vi "Logging Message Loop.vi"(8 "error in (no error)":errorcluster) -> (0 "error out":errorcluster)   [LabVIEW 2020, in "SAVE.lvlib"]
doc: "The message loop subVI to handle messages pertaining to logging data."
uses:
  SAVE.lvlib
  Test Driver/System Preset.ctl
  support/PCT FGV CMD.ctl
  Logging State.ctl
  Save Configuration.ctl
  support/Message Queue/Enqueue Message (Single).vi
  <vilib>/Utility/error.llb/Error Cluster From Error Code.vi
  <vilib>/ErrorRing/Error Ring.xnode
  support/Message Queue/Message Queue.lvlib
panel:
  out "Gage Config":T1(array[cluster])
  out "System Preset":T2 {"Test Configuration"."SP List" format="%#.1g"}
  # "X"
  # "Y"
  # "Cycles"
  # "Point Delay"
  # "Up"
  # "Down"
  # "Z Axes"
  # "#C"
  # "In"
  # "Out"
  # "Cleaning [sec]"
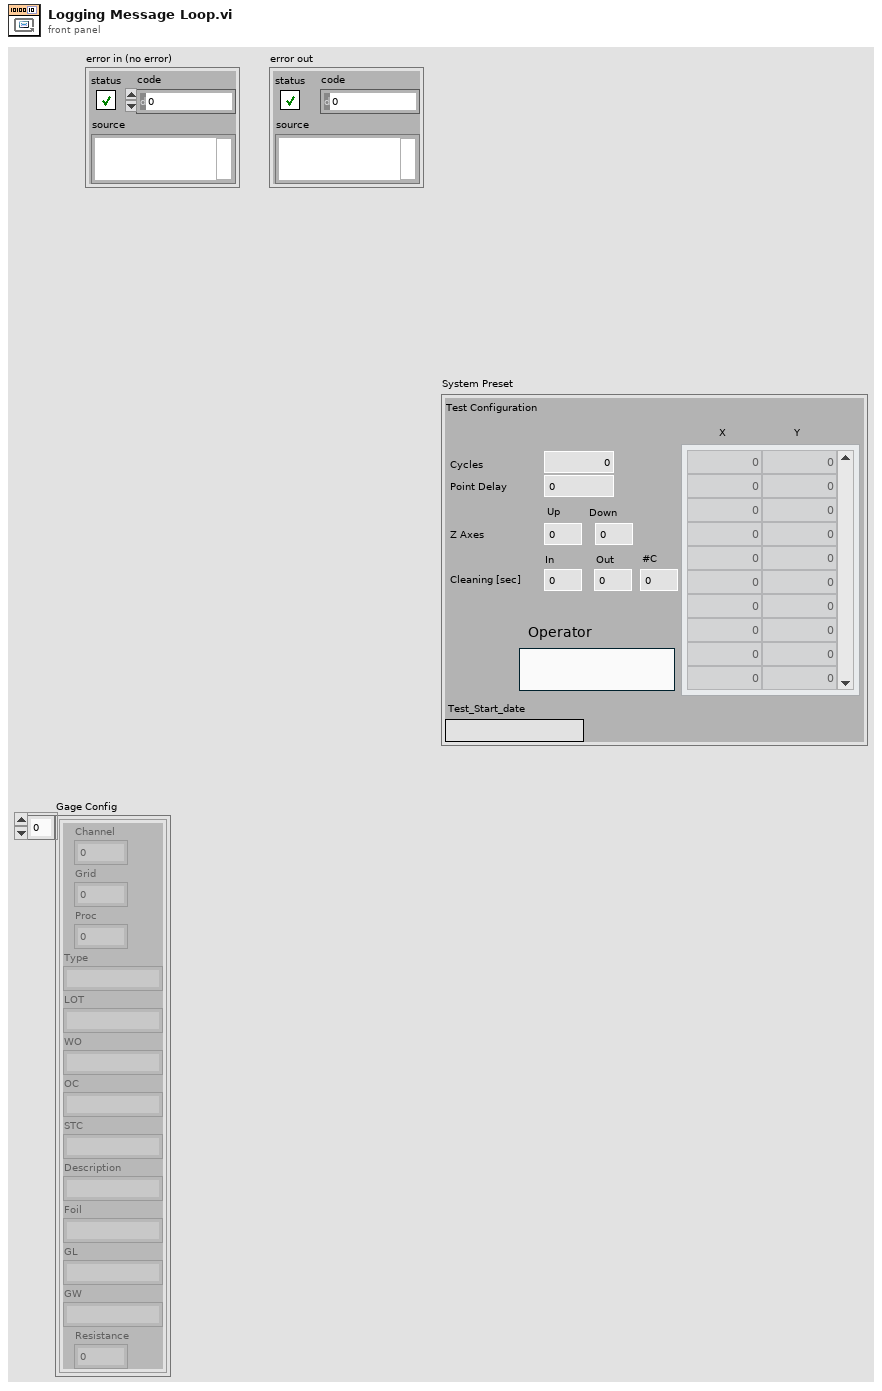
[diagram p1: front panel]
types:
  T1 = cluster{"Channel":u16, "Grid":u16, "Proc":u16, "Type":string, "LOT":string, "WO":string, "OC":string, "STC":string, "Description":string, "Foil":string, "GL":string, "GW":string, "Resistance":dbl}[]
  T2 = typedef "System Preset.ctl" = cluster{"Test Configuration":cluster{"Cycles":i32, "Z Up":dbl, "SP List":dbl[][], "Operator":string, "Point Delay":i32, "Z Up 2":dbl, "Cleaning In":dbl, "Cleaning Out":dbl, "Cleaning Cycles":i32}, "Test_Start_date":string}
  T3 = cluster{"Adhesive Type":string, "Adhesive LOT":string, "Calibration Date":string, "REF Gage Configuration":cluster{"Type":string, "Resistance":dbl, "LOT":string, "Replacement Date":string, "GF":dbl, "Ref Channel":dbl}, "Limits":cluster{"X_t":i32, "X_c":i32, "Exe_t":i32, "Exe_c":i32}, "Gage Config":cluster{"Channel":u16, "Grid":u16, "Proc":u16, "Type":string, "LOT":string, "WO":string, "OC":string, "STC":string, "Description":string, "Foil":string, "GL":string, "GW":string, "Resistance":dbl}[]}
  T4 = typedef "PCT FGV CMD.ctl" = enum16{"INIT", "GET", "SET"}
  T5 = typedef "Message Queue.lvlib/All Message Queues.ctl" = cluster{"UI":refnum<queue>, "Logging":refnum<queue>, "LOG":refnum<queue>, "ALARM":refnum<queue>, "Test":refnum<queue>, "Answer":refnum<queue>, "PLC":refnum<queue>, "DB":refnum<queue>, "Report":refnum<queue>, "OPC":refnum<queue>, "Procedure":refnum<queue>, "PalmSens":refnum<queue>, "SYS 7000 Reader":refnum<queue>, "SWITCH":refnum<queue>, "MOTOR":refnum<queue>, "MOTION":refnum<queue>, "HIDEN":refnum<queue>, "VALVE":refnum<queue>, "MFC":refnum<queue>, "PUMP IN":refnum<queue>, "PUMP OUT":refnum<queue>}
  T6 = typedef "PCT Data REFs.ctl" = cluster{"PLC AI Notifier":refnum<notifier>, "PS Data Queue":refnum<queue>, "BTN Queue":refnum<queue>, "PLC DI notifier":refnum<notifier>, "Timer notifier":refnum<notifier>, "DMM PS":refnum<notifier>, "DMM Gages":refnum<notifier>, "XYZ notifier":refnum<notifier>, "Test Notifier":refnum<notifier>, "Scanner notifier":refnum<notifier>, "OPC Notifier":refnum<notifier>, "HIDEN queue":refnum<queue>}
  T7 = typedef "SAVE.lvlib/Save Configuration.ctl" = cluster{"Log File Base Path":path, "TDMS File Reference":refnum<k34>, "Reset":bool, "Wait":dbl, "Start Time":dbl, "Update Rate":u16, "Channel Names":string[], "System Preset":variant}
  T8 = typedef "SAVE.lvlib/Logging State.ctl" = enum16{"Idle", "Logging"}
  T9 = enum16{"open", "open or create", "create or replace", "create", "open (read-only)"}
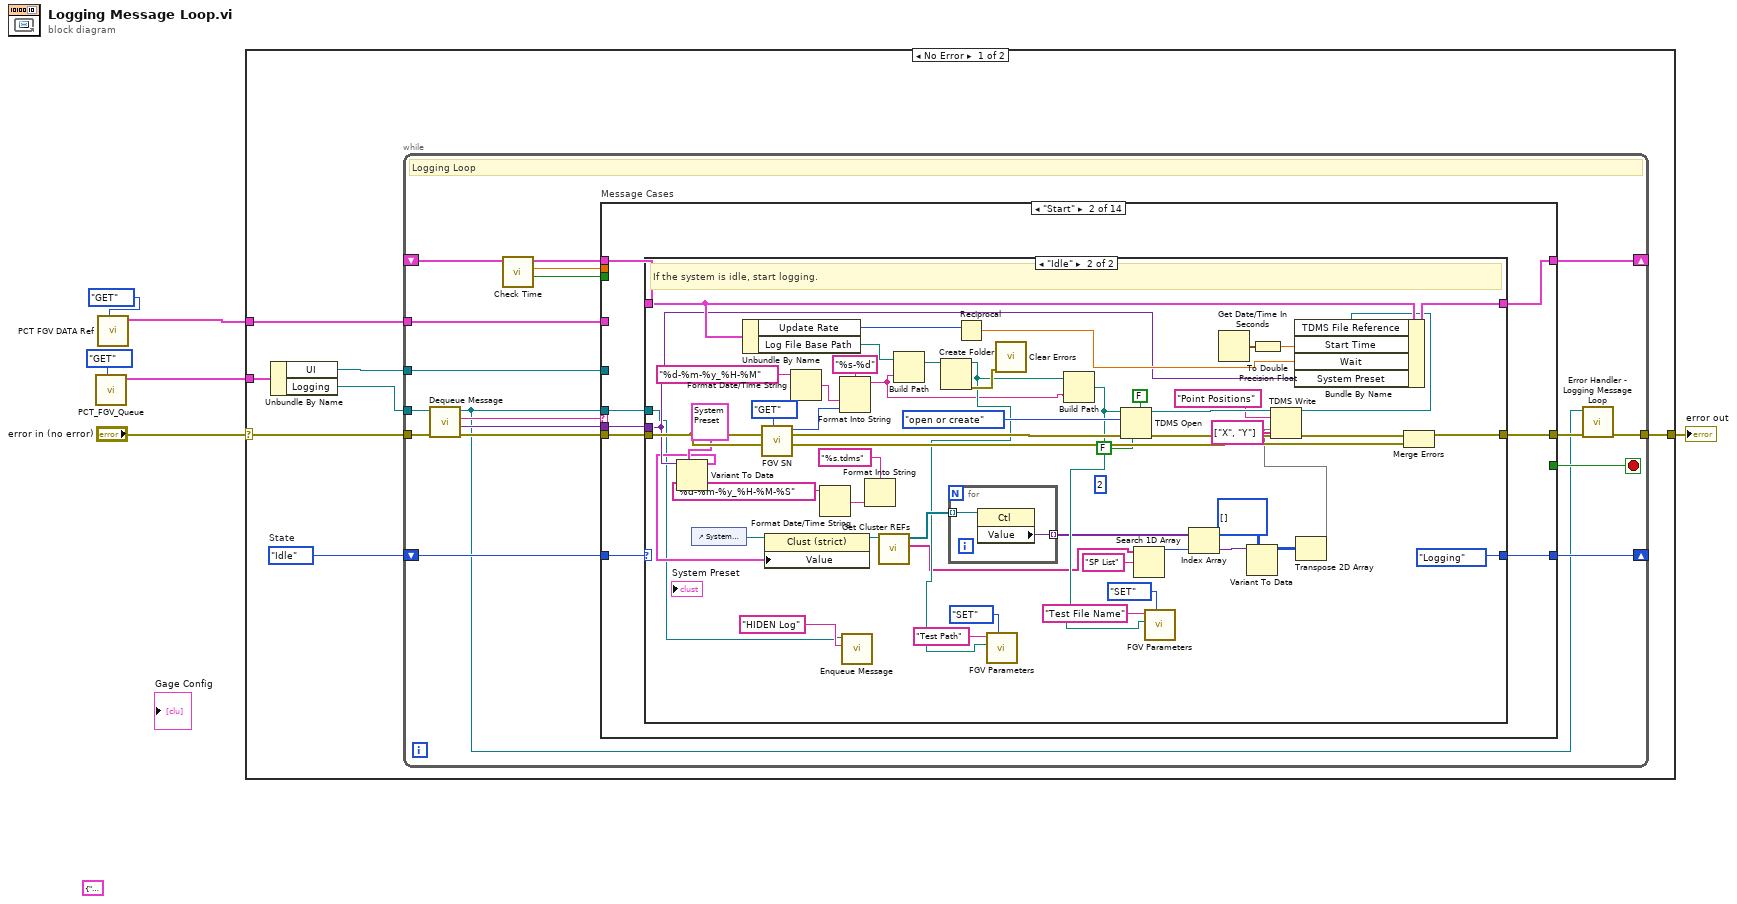
[diagram p0: block diagram]
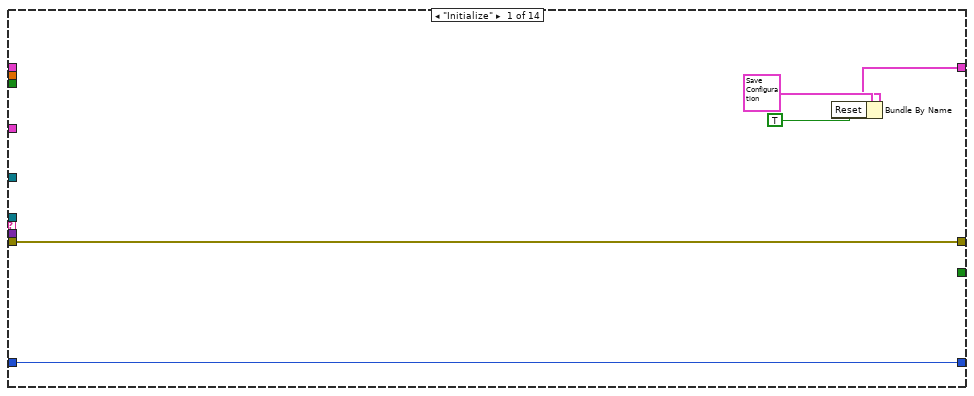
[diagram p2: hidden frame]
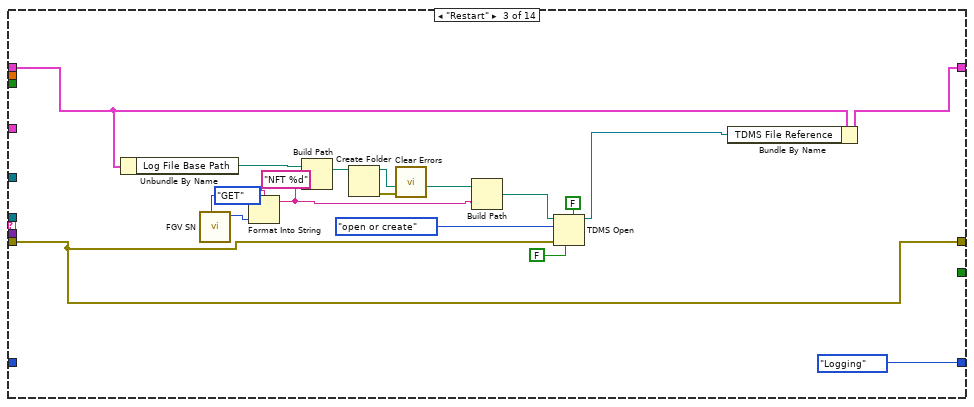
[diagram p4: hidden frame]
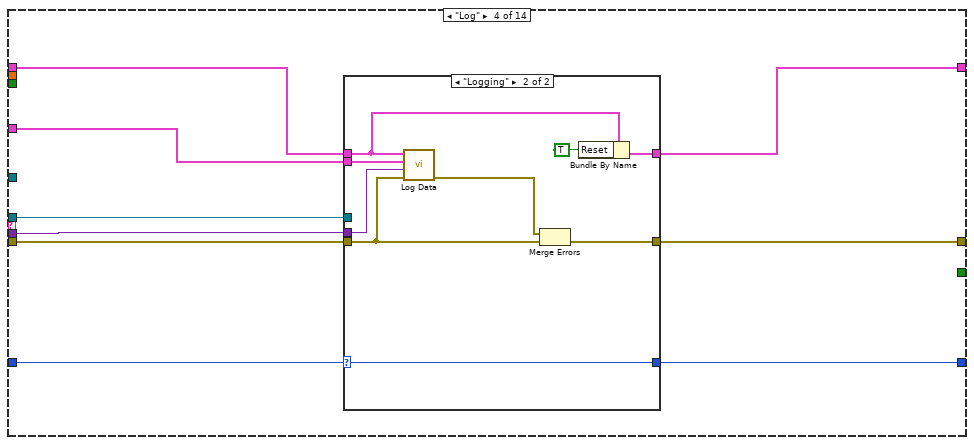
[diagram p5: hidden frame]
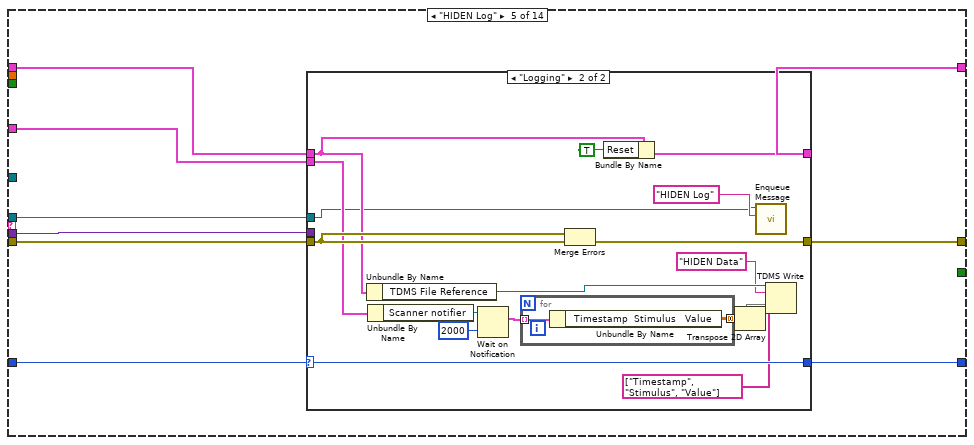
[diagram p7: hidden frame]
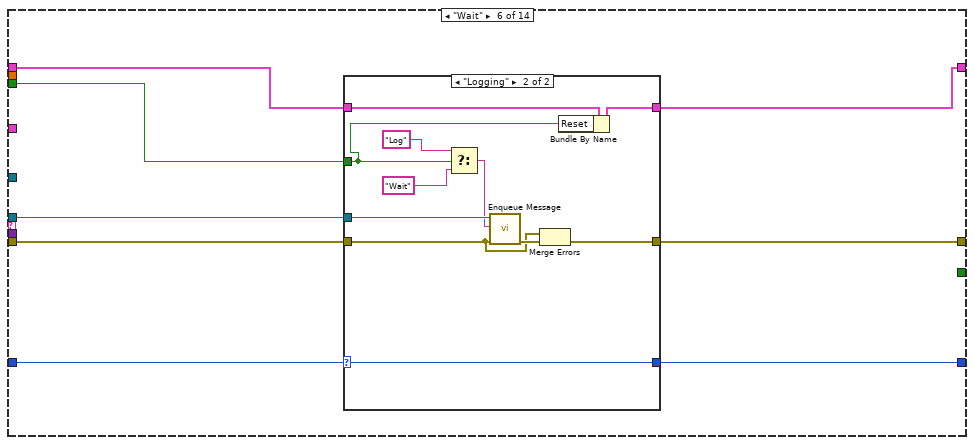
[diagram p9: hidden frame]
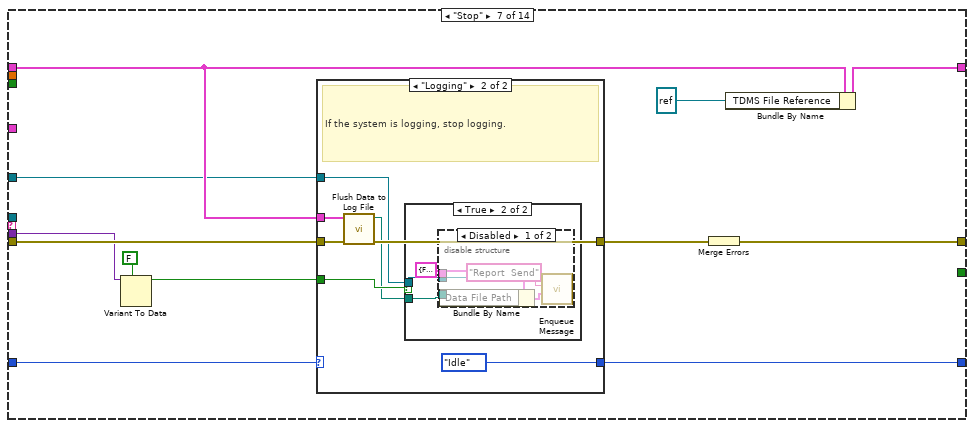
[diagram p11: hidden frame]
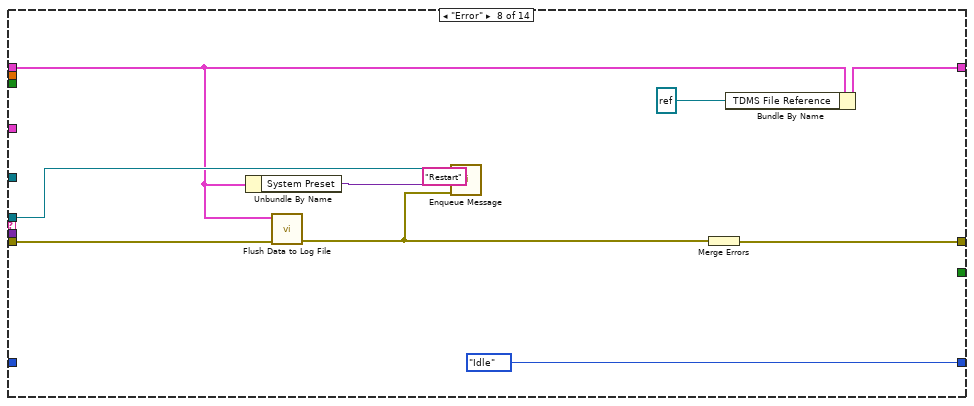
[diagram p15: hidden frame]
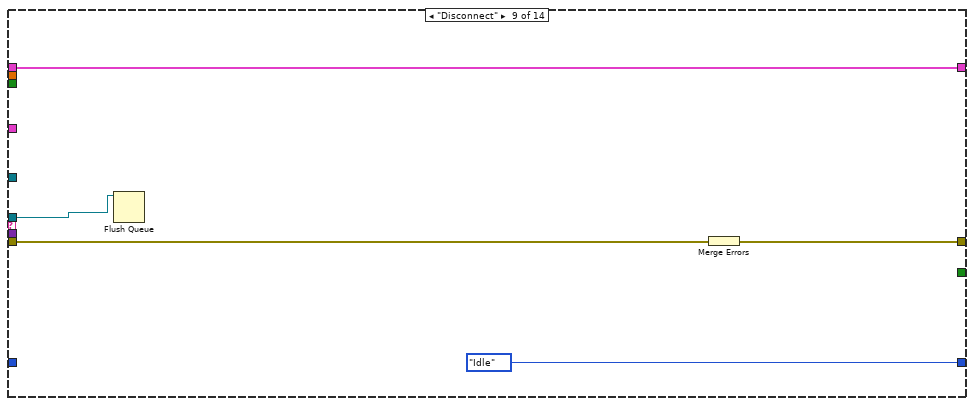
[diagram p16: hidden frame]
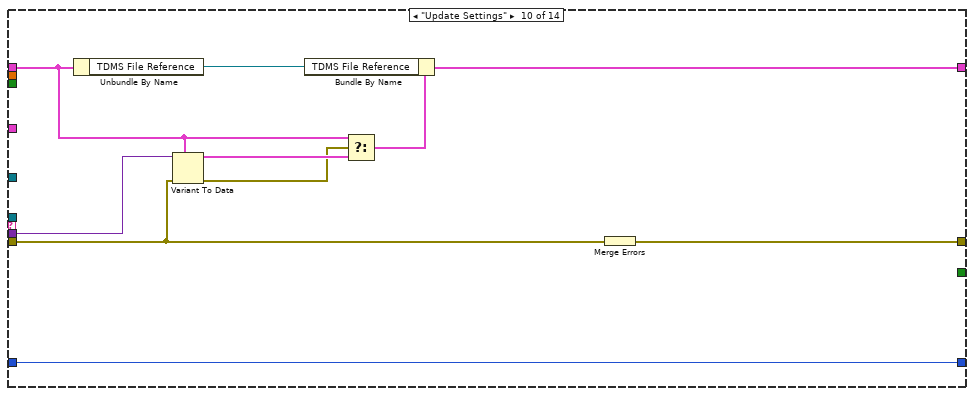
[diagram p17: hidden frame]
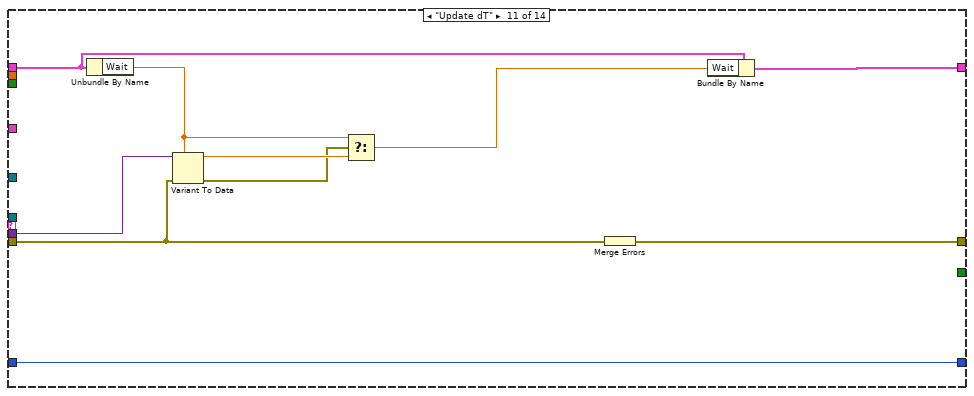
[diagram p18: hidden frame]
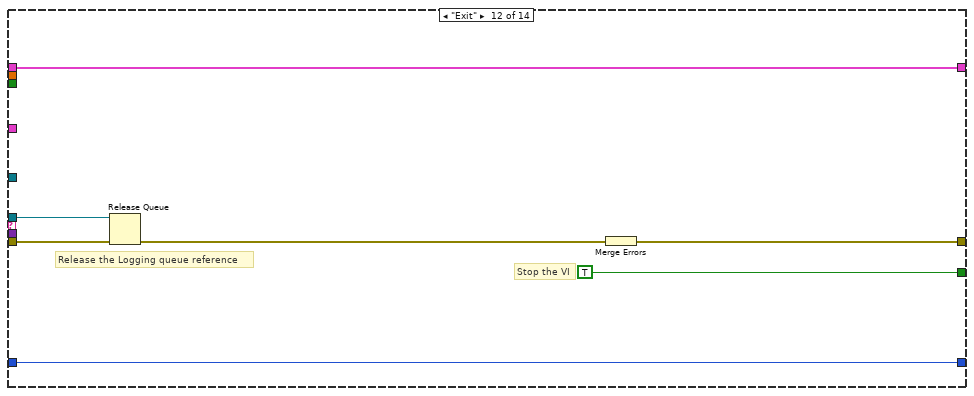
[diagram p19: hidden frame]
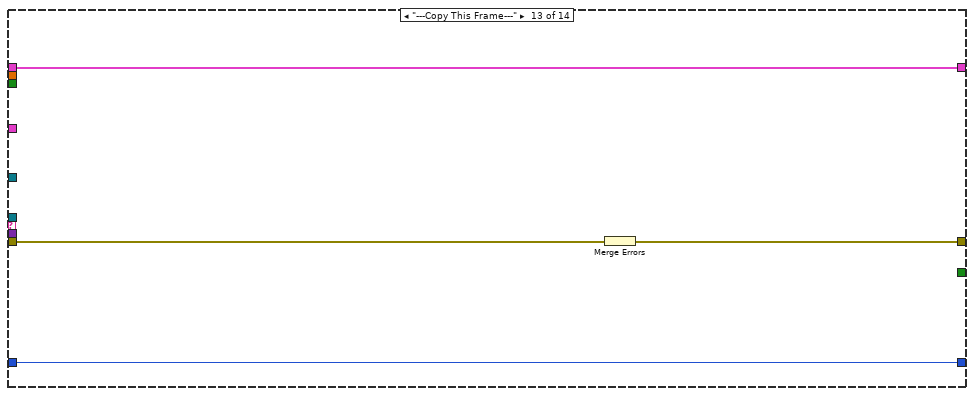
[diagram p20: hidden frame]
diagram:
  (unwired) T3 {"Adhesive Type"="", "Adhesive LOT"="", "Calibration Date"="", "REF Gage Configuration"={"Type"="", "Resistance"=0.0, "LOT"="", "Replacement Date"="", "GF"=0.0, "Ref Channel"=0.0}, "Limits"={"X_t"=0, "X_c"=0, "Exe_t"=0, "Exe_c"=0}, "Gage Config"=[]} ("System Preset")
  n1 = call "PCT_FGV_Queue.vi"("CMD"=PCT_FGV_CMD."GET") -> ("Message Queues out"=w4:T5)  [unwired: 9 in, 1 out]
  n2 = call "PCT FGV DATA Ref.vi"("CMD"=PCT_FGV_CMD."GET") -> ("Data REF"=w1:T6)  [unwired: 9 in, 1 out]
  n3 = case shown="No Error" "error in (no error)" {
    selector: "error in (no error)" -> [w10 w279]
    tunnel: w4 -> [w13 _]
    tunnel: [w11 w279] -> w6
    tunnel: w1 -> [w7 _]
    frame No Error {
      w8 = Logging_State."Idle"  # State
      n4 = Unbundle By Name(w13) -> ("UI"=w9:refnum<queue>, "Logging"=w12:refnum<queue>)
      n5 = while {
        tunnel: w12 -> [w25]
        shift-right: [w31] -> _
        shift-left: _ -> [w19]
        tunnel: w9 -> [w20]
        shift-right: [w23] -> _
        shift-left: w8 -> [w24]
        tunnel: w10 -> [w29]
        tunnel: [w22] -> w11
        tunnel: w7 -> [w15]
        stop <- w30 stop-if-true
        # "Logging Loop"
        n6 = call "Dequeue Message.vi"("error in (no error)"=w29, "Message Queue"=w25) -> ("error out"=w28:errorcluster, "Message Data"=w26:variant, "Message"=w27:string, "dup Message Queue"=w14:refnum<queue>)  [unwired: 6 in]
        n7 = call "Check Time.vi"("Logging Configuration"=w19) -> ("Time has Elapsed"=w16:bool, "Elapsed Time (s)"=w17:dbl, "Logging Configuration out"=w18:T7)  [unwired: 8 in]
        n8 = case "Message Cases" shown="\"Start\"" w27 {
          selector: w27 -> [_ _ _ _ _ _ _ _ _ _ _ _ _ w268]
          tunnel: w14 -> [_ w43 _ w126 w147 w177 _ w226 w232 _ _ w260 _ _]
          tunnel: w28 -> [w36 w42 w118 w125 w146 w176 w199 w228 w234 w241 w252 w261 w267 _]
          tunnel: [w36 w44 w118 w127 w148 w178 w204 w231 w236 w246 w256 w262 w265 w269] -> w21
          tunnel: w18 -> [_ w41 w117 w121 w142 w172 w200 w224 w235 w238 w247 w258 w266 w271]
          tunnel: [w33 w40 w116 w120 w141 w171 w202 w230 w235 w239 w248 w258 w266 w271] -> w31
          tunnel: [_ _ _ _ _ _ _ _ _ _ _ TRUE _ _] -> w30
          tunnel: w26 -> [_ w37 _ w119 w140 _ w195 _ _ w245 w255 _ _ _]
          tunnel: w20 -> [_ _ _ _ _ _ w196 _ _ _ _ _ _ _]
          tunnel: w24 -> [w35 w39 _ w124 w145 w175 w198 _ _ w240 w251 w257 w264 w270]
          tunnel: [w35 w38 Logging_State."Logging" ("State") w123 w144 w174 w197 Logging_State."Idle" ("State") Logging_State."Idle" ("State") w240 w251 w257 w264 w270] -> w23
          tunnel: w17 -> [_ _ _ _ _ _ _ _ _ _ _ _ _ _]
          tunnel: w16 -> [_ _ _ _ _ w173 _ _ _ _ _ _ _ _]
          tunnel: w15 -> [_ _ _ w122 w143 _ _ _ _ _ _ _ _ _]
          frame "Initialize" {
            # "Initialize - gets called when first launched. Currently a no-op."
            n9 = Bundle By Name(cluster=T7 {"Log File Base Path"=path "", "TDMS File Reference"=refnum, "Reset"=FALSE, "Wait"=0.0, "Start Time"=0.0, "Update Rate"=1, "Channel Names"=[], "System Preset"=variant} ("Logging Configuration"), "Reset"=TRUE) -> (w33:T7)
          }
          frame "Start" {
            # "Start - Send the \"Log\" message to start logging.  Generate a unique, timestamped TDMS file name based on the Log File Base Path value."
            n10 = case shown="\"Idle\"" w39 {
              selector: w39 -> [w46 _]
              tunnel: [w45 w95] -> w44
              tunnel: w43 -> [_ w49]
              tunnel: w42 -> [w45 w94]
              tunnel: w41 -> [w47 w96]
              tunnel: [w47 w98] -> w40
              tunnel: [w46 Logging_State."Logging" ("State")] -> w38
              tunnel: w37 -> [_ w67]
              frame "Logging" {
                # "The system is already logging. Ignore the \"Start\" message."
              }
              frame "Idle" {
                (unwired) 2 ("length")
                # "If the system is idle, start logging."
                n11 = Variant To Data(type=T2 {"Test Configuration"={"Cycles"=0, "Z Up"=0.0, "SP List"=[], "Operator"="", "Point Delay"=0, "Z Up 2"=0.0, "Cleaning In"=0.0, "Cleaning Out"=0.0, "Cleaning Cycles"=0}, "Test_Start_date"=""} ("System Preset"), Variant=w67) -> (data=w63:T2)  [unwired: 1 in, 1 out]
                n12 = control-ref of="System Preset"() -> (w48:refnum<vi>)
                n13 = Unbundle By Name(w96) -> ("Update Rate"=w88:u16, "Log File Base Path"=w79:path)
                n14 = call "FGV SN.vi"("CMD"=PCT_FGV_CMD."GET") -> ("output"=w65:i32)  [unwired: 9 in, 1 out]
                n15 = property class="Clust (strict)"(reference=w48, "Value"=w63) -> (reference out=w81:refnum<vi>)  [unwired: 1 in, 1 out]
                n16 = Format Date/Time String(time format string (%c)="%d-%m-%y_%H-%M") -> (date/time string=w51:string)  [unwired: 2 in]
                n17 = Format Date/Time String(time format string (%c)="%d-%m-%y_%H-%M-%S") -> (date/time string=w73:string)  [unwired: 2 in]
                n18 = Format Into String(format string="%s-%d", w51, w65) -> (resulting string=w64:string)  [unwired: 2 in, 1 out]
                n19 = call-poly "Enqueue Message.vi"("Message"="HIDEN Log" ("time format string (%c)"), "Message Queue"=w49) -> ()  [unwired: 8 in, 2 out]
                n20 = Format Into String(format string="%s.tdms", w73) -> ()  [unwired: 2 in, 2 out]
                n21 = call "Get Cluster REFs.vi"("Cluster in"=w81) -> ("Names"=w62:string[], "controls[]"=w83:refnum<vi>[])  [unwired: 8 in, 1 out]
                n22 = Build Path(base path=w79, name or relative path=w64) -> (appended path=w78:path)
                n23 = Create Folder(path (use dialog)=w78) -> (created path=w74:path, error out=w77:errorcluster)  [unwired: 2 in, 1 out]
                n24 = for {
                  tunnel: w83 -> [w101] mode=indexing
                  tunnel: [w100] -> w60 mode=indexing
                  n25 = property class="Ctl"(reference=w101) -> ("Value"=w100:variant)  [unwired: 1 in, 2 out]
                }
                n26 = Reciprocal(x=w88) -> (1/x=w87:dbl)
                n27 = call "FGV Parameters.vi"("CMD"=PCT_FGV_CMD."SET", "input"=w74, "Key"="Test Path") -> ()  [unwired: 6 in, 3 out]
                n28 = call <vilib>:"Clear Errors.vi"("error in (no error)"=w77) -> ()  [unwired: 5 in, 2 out]
                n29 = Build Path(base path=w74, name or relative path=w64) -> (appended path=w69:path)
                n30 = TDMS Open(5:FALSE ("create index file? (T)"), 6:FALSE ("disable buffering? (T)"), 8:w94, 10:T9."open or create" ("operation (0:open)"), 11:w69) -> (0:w91:errorcluster, 3:w89:refnum<k34>)  [unwired: 2 in]
                n31 = Search 1D Array(1D array=w62, element="SP List") -> (index of element=w59:i32)  [unwired: 1 in]
                n32 = call "FGV Parameters.vi"("CMD"=PCT_FGV_CMD."SET", "input"=w69, "Key"="Test File Name") -> ()  [unwired: 6 in, 3 out]
                n33 = Index Array(array=w60, index=w59) -> (element=w58:variant)
                n34 = Get Date/Time In Seconds() -> (seconds since 1Jan1904=w93:timestamp)
                n35 = Variant To Data(type=i32[][] [], Variant=w58) -> (data=w55:i32[][])  [unwired: 1 in, 1 out]
                n36 = To Double Precision Float(number=w93) -> (double precision float=w92:dbl)
                n37 = Transpose 2D Array(2D array=w55) -> (transposed array=w53:i32[][])
                n38 = TDMS Write(0:w89, 5:"Point Positions" ("group name in (Untitled)"), 7:string[] ["X", "Y"] ("channel name(s) in (Untitled)"), 9:w53, 11:w91) -> (4:w80:refnum<k34>, 15:w90:errorcluster)  [unwired: 1 in, 2 out]
                n39 = Bundle By Name(cluster=w96, "TDMS File Reference"=w80, "Start Time"=w92, "Wait"=w87, "System Preset"=w67) -> (w98:T7)
                n40 = Merge Errors(w90, w94) -> (w95:errorcluster)
              }
            }
          }
          frame "Restart" {
            # "Start - Send the \"Log\" message to start logging.  Generate a unique, timestamped TDMS file name based on the Log File Base Path value."
            n41 = Unbundle By Name(w117) -> ("Log File Base Path"=w112:path)
            n42 = call "FGV SN.vi"("CMD"=PCT_FGV_CMD."GET") -> ("output"=w104:i32)  [unwired: 9 in, 1 out]
            n43 = Format Into String(format string="NFT %d", w104) -> (resulting string=w103:string)  [unwired: 2 in, 1 out]
            n44 = Build Path(base path=w112, name or relative path=w103) -> (appended path=w111:path)
            n45 = Create Folder(path (use dialog)=w111) -> (created path=w109:path, error out=w110:errorcluster)  [unwired: 2 in, 1 out]
            n46 = call <vilib>:"Clear Errors.vi"("error in (no error)"=w110) -> ()  [unwired: 5 in, 2 out]
            n47 = Build Path(base path=w109, name or relative path=w103) -> (appended path=w107:path)
            n48 = TDMS Open(5:FALSE ("create index file? (T)"), 6:FALSE ("disable buffering? (T)"), 8:w118, 10:T9."open or create" ("operation (0:open)"), 11:w107) -> (3:w102:refnum<k34>)  [unwired: 2 in, 1 out]
            n49 = Bundle By Name(cluster=w117, "TDMS File Reference"=w102) -> (w116:T7)
          }
          frame "Log" {
            # "Log - Log data to disk. Since this is a continuous acquisition, this message will always message itself to run again."
            n50 = case shown="\"Logging\"" w124 {
              selector: w124 -> [w130 w136]
              tunnel: [w129 w139] -> w127
              tunnel: w126 -> [_ _]
              tunnel: w122 -> [_ w138]
              tunnel: w125 -> [w129 w135]
              tunnel: w121 -> [w128 w134]
              tunnel: [w130 w136] -> w123
              tunnel: [w128 w132] -> w120
              tunnel: w119 -> [_ w131]
              frame "Idle" {
                # "Ignore \"Log\" messages when the logging is idle."
              }
              frame "Logging" {
                # "Log more data while in the \"Logging\" state."
                n51 = call "Log Data.vi"("error in (no error)"=w135, "variant"=w131, "Data REF"=w138, "Logging Configuration"=w134) -> ("error out"=w137:errorcluster)  [unwired: 7 in]
                n52 = Merge Errors(w137, w135) -> (w139:errorcluster)
                n53 = Bundle By Name(cluster=w134, "Reset"=TRUE) -> (w132:T7)
              }
            }
          }
          frame "HIDEN Log" {
            # "Log - Log data to disk. Since this is a continuous acquisition, this message will always message itself to run again."
            n54 = case shown="\"Logging\"" w145 {
              selector: w145 -> [w151 w167]
              tunnel: [w150 w168] -> w148
              tunnel: w147 -> [_ w154]
              tunnel: w143 -> [_ w163]
              tunnel: w146 -> [w150 w166]
              tunnel: w142 -> [w149 w162]
              tunnel: [w151 w167] -> w144
              tunnel: [w149 w164] -> w141
              tunnel: w140 -> [_ _]
              frame "Idle" {
                # "Ignore \"Log\" messages when the logging is idle."
              }
              frame "Logging" {
                # "Log more data while in the \"Logging\" state."
                n55 = Unbundle By Name(w162) -> ("TDMS File Reference"=w161:refnum<k34>)
                n56 = Unbundle By Name(w163) -> ("Scanner notifier"=w160:refnum<notifier>)
                n57 = Wait on Notification(notifier=w160, timeout in ms (-1)=2000) -> (notification=w159:cluster{"Timestamp  Stimulus   Value":dbl[][]}[])  [unwired: 2 in, 3 out]
                n58 = for {
                  tunnel: w159 -> [w170] mode=indexing
                  tunnel: [w169] -> w158 mode=concatenating
                  n59 = Unbundle By Name(w170) -> ("Timestamp  Stimulus   Value"=w169:dbl[][])
                }
                n60 = Merge Errors(w166, w166) -> (w168:errorcluster)
                n61 = Bundle By Name(cluster=w162, "Reset"=TRUE) -> (w164:T7)
                n62 = Transpose 2D Array(2D array=w158) -> (transposed array=w152:dbl[][])
                n63 = call-poly "Enqueue Message.vi"("Message"="HIDEN Log" ("time format string (%c)"), "Message Queue"=w154) -> ()  [unwired: 8 in, 2 out]
                n64 = TDMS Write(0:w161, 5:"HIDEN Data" ("group name in (Untitled)"), 7:string[] ["Timestamp", "Stimulus", "Value"] ("channel name(s) in (Untitled)"), 9:w152) -> ()  [unwired: 2 in, 4 out]
              }
            }
          }
          frame "Wait" {
            # "Log - Log data to disk. Since this is a continuous acquisition, this message will always message itself to run again."
            n65 = case shown="\"Logging\"" w175 {
              selector: w175 -> [w181 w189]
              tunnel: [w180 w192] -> w178
              tunnel: w177 -> [_ w190]
              tunnel: w176 -> [w180 w188]
              tunnel: [w181 w189] -> w174
              tunnel: w173 -> [_ w182]
              tunnel: w172 -> [w179 w184]
              tunnel: [w179 w183] -> w171
              frame "Idle" {
                # "Ignore \"Log\" messages when the logging is idle."
              }
              frame "Logging" {
                # "Log more data while in the \"Logging\" state."
                n66 = Select(t="Log" ("Message"), s=w182, f="Wait" ("Message")) -> (s? t:f=w186:string)
                n67 = call-poly "Enqueue Message.vi"("error in (no error)"=w188, "Message"=w186, "Message Queue"=w190) -> ("error out"=w191:errorcluster)  [unwired: 7 in, 1 out]
                n68 = Merge Errors(w188, w191) -> (w192:errorcluster)
                n69 = Bundle By Name(cluster=w184, "Reset"=w182) -> (w183:T7)
              }
            }
          }
          frame "Stop" {
            # "Stop - Flush the message queue of any pending \"Log\" messages. Call 'Flush Data to Log File.vi' so any pending data is not lost."
            n70 = Variant To Data(type=FALSE, Variant=w195) -> (data=w193:bool)  [unwired: 1 in, 1 out]
            n71 = case shown="\"Logging\"" w198 {
              selector: w198 -> [w205 _]
              tunnel: [w206 w210] -> w203
              tunnel: w200 -> [_ w213]
              tunnel: w199 -> [w206 w212]
              tunnel: [w205 Logging_State."Idle" ("State")] -> w197
              tunnel: w196 -> [_ w208]
              tunnel: w193 -> [_ w209]
              frame "Idle" {
                # "The system is already idle. Ignore the \"Stop\" message."
              }
              frame "Logging" {
                # "If the system is logging, stop logging."
                n72 = call "Flush Data to Log File.vi"("error in (no error)"=w212, "Logging Configuration"=w213) -> ("error out"=w210:errorcluster, "file path out"=w207:path)  [unwired: 8 in]
                n73 = case shown="True" w209 {
                  tunnel: w208 -> [_ w216]
                  tunnel: w207 -> [_ w214]
                  frame False {
                  }
                  frame True {
                    n74 = disable-structure shown="Disabled" {
                      disable-tunnel: w216 -> [w221 _]
                      disable-tunnel: cluster{bool, "Data File Path":path} {FALSE, "Data File Path"=path ""} -> [w219 _]
                      disable-tunnel: w214 -> [w217 _]
                      frame Disabled {
                        n75 = Bundle By Name(cluster=w219, "Data File Path"=w217) -> (w218:cluster{bool, "Data File Path":path})
                        n76 = call-poly "Enqueue Message.vi"("Message Data"=w218, "Message"="Report  Send", "Message Queue"=w221) -> ()  [unwired: 7 in, 2 out]
                      }
                      frame Enabled {
                      }
                    }
                  }
                }
              }
            }
            n77 = Merge Errors(w203) -> (w204:errorcluster)
            n78 = Bundle By Name(cluster=w200, "TDMS File Reference"=refnum<k34> refnum) -> (w202:T7)
          }
          frame "Error" {
            # "Stop - Flush the message queue of any pending \"Log\" messages. Call 'Flush Data to Log File.vi' so any pending data is not lost."
            n79 = Unbundle By Name(w224) -> ("System Preset"=w223:variant)
            n80 = call "Flush Data to Log File.vi"("error in (no error)"=w228, "Logging Configuration"=w224) -> ("error out"=w225:errorcluster)  [unwired: 8 in, 1 out]
            n81 = call-poly "Enqueue Message.vi"("error in (no error)"=w225, "Message Data"=w223, "Message"="Restart", "Message Queue"=w226) -> ()  [unwired: 6 in, 2 out]
            n82 = Merge Errors(w225) -> (w231:errorcluster)
            n83 = Bundle By Name(cluster=w224, "TDMS File Reference"=refnum<k34> refnum) -> (w230:T7)
          }
          frame "Disconnect" {
            # "Stop - Flush the message queue of any pending \"Log\" messages. Call 'Flush Data to Log File.vi' so any pending data is not lost."
            n84 = Flush Queue(queue=w232) -> ()  [unwired: 1 in, 3 out]
            n85 = Merge Errors(w234) -> (w236:errorcluster)
          }
          frame "Update Settings" {
            # "Update Settings - New settings are available, update the current ones stored in the shift register with the settings sent as part of the message."
            n86 = Unbundle By Name(w238) -> ("TDMS File Reference"=w237:refnum<k34>)
            n87 = Variant To Data(error in=w241, type=w238, Variant=w245) -> (data=w244:T7, error out=w243:errorcluster)
            n88 = Select(t=w238, s=w243, f=w244) -> (s? t:f=w242:T7)
            n89 = Bundle By Name(cluster=w242, "TDMS File Reference"=w237) -> (w239:T7)
            n90 = Merge Errors(w241) -> (w246:errorcluster)
          }
          frame "Update dT" {
            # "Update Settings - New settings are available, update the current ones stored in the shift register with the settings sent as part of the message."
            n91 = Unbundle By Name(w247) -> ("Wait"=w250:dbl)
            n92 = Variant To Data(error in=w252, type=w250, Variant=w255) -> (data=w254:dbl, error out=w253:errorcluster)
            n93 = Select(t=w250, s=w253, f=w254) -> (s? t:f=w249:dbl)
            n94 = Merge Errors(w252) -> (w256:errorcluster)
            n95 = Bundle By Name(cluster=w247, "Wait"=w249) -> (w248:T7)
          }
          frame "Exit" {
            # "Release the Logging queue reference"
            # "Stop the VI"
            # "Exit - Send the Exit message to the UI Message Handler.  Call 'Flush Data to Log File.vi' so any pending data is not lost."
            n96 = Release Queue(queue=w260, error in (no error)=w261) -> (error out=w259:errorcluster)  [unwired: 1 in, 2 out]
            n97 = Merge Errors(w259) -> (w262:errorcluster)
          }
          frame "---Copy This Frame---" {
            # "Duplicate this frame when creating new messages.  Change this comment in the duplicated frame to describe this message."
            n98 = Merge Errors(w267) -> (w265:errorcluster)
          }
          frame Default {
            # "'Default' case only runs if there is a message that isn't defined in any of the other cases.  Output a programming error."
            n99 = xnode "Error Ring"("parameter 0"=w268) -> ("error out"=w269:errorcluster)
          }
        }
        n100 = call "Error Handler - Logging Message Loop.vi"("error in (no error)"=w21, "Message Queue"=w14) -> ("dup error in"=w22:errorcluster)  [unwired: 8 in, 1 out]
      }
    }
    frame Error {
    }
  }
  "error out" <- w6
